vi "vetores_girada.vi"(7 "Raio":dbl=123.0, 8 "Target":dbl[](array[numeric]), 9 "Target 2":dbl[](array[numeric]), 10 "Robot in":refnum<class "Robot.lvclass">=refnum, 11 "Game in":refnum<class "Game.lvclass">=refnum) -> (0 "Norm RB":dbl format="%0.2f", 1 "Norm TR":dbl format="%0.2f", 2 "Versor R->B":dbl[](array[numeric]) format="%0.2f", 3 "Versor T->R":dbl[](array[numeric]) format="%0.2f", 4 "Norm TB":dbl format="%0.2f", 5 "Versor T->B":dbl[](array[numeric]) format="%0.2f", 6 "robo position in circle location":dbl[](array[numeric]))   [LabVIEW 2021]
uses:
  Game_class/Game.lvclass
  Robot_class/Robot.lvclass
  C:/Users/IME/Desktop/Horie - VSS - SSL/SSL_AI/Object_class/Object.lvclass
  Ally_class/Ally.lvclass
  Ball_class/Ball.lvclass
  Referee_class/Referee.lvclass
  Field_class/Field.lvclass
  Enemy_class/Enemy.lvclass
  Events_class/Events.lvclass
  Utilities_class/Utilities.lvclass
  Parameters_class/Parameters.lvclass
  Playbook_class/Playbook.lvclass
  Play_class/Play.lvclass
  TestPlay_class/TestPlay.lvclass
  EnemyPossessionAtEnemyFieldPlay_class/EnemyPossessionAtEnemyFieldPlay.lvclass
  EnemyPossessionAtOurFieldPlay_class/EnemyPossessionAtOurFieldPlay.lvclass
  NormalGamePlay_class/NormalGamePlay.lvclass
  IndirectEnemyPlay_class/IndirectEnemyPlay.lvclass
  PrepareKickoffAllyPlay_class/PrepareKickoffAllyPlay.lvclass
  PrepareKickoffEnemyPlay_class/PrepareKickoffEnemyPlay.lvclass
  KickPenaltyAllyPlay_class/KickPenaltyAllyPlay.lvclass
  PreparePenaltyAllyPlay_class/PreparePenaltyAllyPlay.lvclass
  DirectEnemyPlay_class/DirectEnemyPlay.lvclass
  PreparePenaltyEnemyPlay_class/PreparePenaltyEnemyPlay.lvclass
  BallOutOfFieldPlay_class/BallOutOfFieldPlay.lvclass
  StopOffensivePlay_class/StopOffensivePlay.lvclass
  PassPlay_class/PassPlay.lvclass
  DirectKickPlay_class/DirectKickPlay.lvclass
  HaltPlay_class/HaltPlay.lvclass
  PreparePassPlay_class/PreparePassPlay.lvclass
  PassToStriker_class/PassToStriker.lvclass
  PassTo2ndStriker_class/PassTo2ndStriker.lvclass
  SimplePass_class/SimplePass.lvclass
  PrepareRollToPassPlay_class/PrepareRollToPassPlay.lvclass
  PrepareDoublePassPlay_class/PrepareDoublePassPlay.lvclass
  TableWith2ndStrikerPlay_class/TableWith2ndStrikerPlay.lvclass
  TableWithStrikerPlay_class/TableWithStrikerPlay.lvclass
  PrepareTriplePassPlay_class/PrepareTriplePassPlay.lvclass
  ABCPassPlay_class/ABCPassPlay.lvclass
  PreparePassInGame1_class/PreparePassInGame1.lvclass
  ACBPassPlay_class/ACBPassPlay.lvclass
  PrepareKeeperPassPlay_class/PrepareKeeperPassPlay.lvclass
  KeeperPassToStrikerPlay_class/KeeperPassToStrikerPlay.lvclass
  5RobotsNormalGamePlay_class/5RobotsNormalGamePlay.lvclass
  Rolebook_class/Rolebook.lvclass
  5RobotsRole_class/5RobotsRole.lvclass
  Tacticbook_class/Tacticbook.lvclass
  ShootRole_class/ShootRole.lvclass
  5RobotsPassGamePlay_class/5RobotsPassGamePlay.lvclass
  PassBestRobotRole_class/PassBestRobotRole.lvclass
  PassBestReceiverRole_class/PassBestReceiverRole.lvclass
  5RobotsKeeperGame_class/5RobotsKeeperGame.lvclass
  5PreparePassGamePlay_class/5PreparePassGamePlay.lvclass
  NormalDefensivePlay_class/NormalDefensivePlay.lvclass
  NormalDefensiveWithDuelistPlay_class/NormalDefensiveWithDuelistPlay.lvclass
  KeeperPlay_class/KeeperPlay.lvclass
  KeeperRole_class/KeeperRole.lvclass
  TimeoutPlay_class/TimeoutPlay.lvclass
  ZigZagPlay_class/ZigZagPlay.lvclass
  GoToPlay_class/GoToPlay.lvclass
  BallPlacementPlay_class/BallPlacementPlay.lvclass
  BallPlacementAllyPlay_class/BallPlacementAllyPlay.lvclass
  SimpleBallPlacementAllyPlay_class/SimpleBallPlacementAllyPlay.lvclass
  RobotFeedback/RobotFeedback.lvclass
  Game_class/Game.lvclass/Game.ctl
  Object_class/Object.lvclass/Object.ctl
  <vilib>/Analysis/baseanly.llb/Unit Vector (DBL).vi
  Object_class/Read position(x,y).vi
  Game_class/Read BallRef.vi
  <vilib>/Analysis/NI_AALBase.lvlib
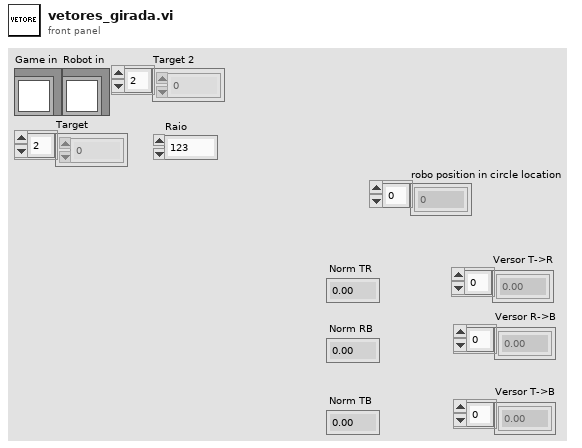
[diagram p1: front panel]
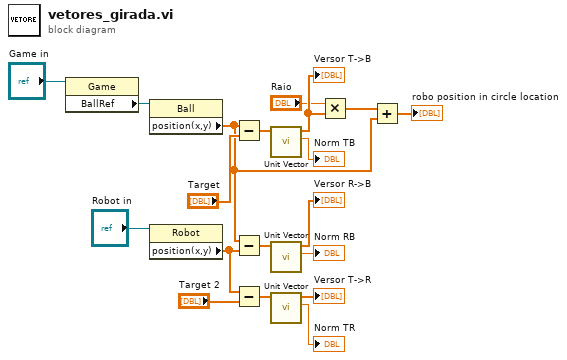
[diagram p0: block diagram]
diagram:
  n1 = property class="Game"(reference="Game in") -> ("BallRef"=w17:refnum<class "Ball.lvclass">)  [unwired: 1 in, 2 out]
  n2 = property class="Ball"(reference=w17) -> ("position(x,y)"=w2:dbl[])  [unwired: 1 in, 2 out]
  n3 = property class="Robot"(reference="Robot in") -> ("position(x,y)"=w14:dbl[])  [unwired: 1 in, 2 out]
  n4 = Subtract(x=w2, y="Target") -> (x-y=w13:dbl[])
  n5 = Subtract(x=w2, y=w14) -> (x-y=w16:dbl[])
  n6 = Subtract(x=w14, y="Target 2") -> (x-y=w15:dbl[])
  n7 = call-poly <vilib>:"Unit Vector.vi"("Input Vector"=w13) -> ("norm"=→"Norm TB":dbl, "Unit Vector"=w5:dbl[])  [unwired: 8 in, 1 out]
  "Versor T->B" <- w5
  n8 = call-poly <vilib>:"Unit Vector.vi"("Input Vector"=w16) -> ("norm"=→"Norm RB":dbl, "Unit Vector"=→"Versor R->B":dbl[])  [unwired: 8 in, 1 out]
  n9 = call-poly <vilib>:"Unit Vector.vi"("Input Vector"=w15) -> ("norm"=→"Norm TR":dbl, "Unit Vector"=→"Versor T->R":dbl[])  [unwired: 8 in, 1 out]
  n10 = Multiply(x="Raio", y=w5) -> (x*y=w3:dbl[])
  n11 = Add(x=w3, y=w2) -> (x+y=→"robo position in circle location":dbl[])
